vi "calc com end of volume.vi"(10 "end of volume":bool, 11 "running sums in":T1) -> (0 "ready for input":bool, 1 "output valid":bool, 2 "center of mass":cluster{"x avg":i16, "y avg":i16, "z avg":i16}, 3 "running sums out":T1, 5 "running sums eov":T1)   [LabVIEW 2010]
uses:
  <vilib>/rvi/FXPMathLib/FxpReciprocal/XNode/nifxpmath_Reciprocal.xnode
  <vilib>/rvi/FXPMathLib/FxpDiv/XNode/nifxpmath_Div.xnode
  <vilib>/rvi/FXPMathLib/FxpDiv/subVIs/nifxpmath_Div_SimConfig.ctl
  <vilib>/rvi/FXPMathLib/FxpMul/XNode/nifxpmath_Multiplier.xnode
  <vilib>/rvi/FXPMathLib/FxpMul/subVIs/nifxpmath_Mul_SimConfig.ctl
  <vilib>/fxp/LVFixedPointQuantizationPolicyTypeDef.ctl
  <vilib>/fxp/LVFixedPointOverflowPolicyTypeDef.ctl
  <vilib>/rvi/FXPMathLib/FxpDiv/simVIs/DllFxpDivTemp_sub.vi
  <vilib>/rvi/FXPMathLib/FxpMul/simVIs/DllFxpMulTemp_sub.vi
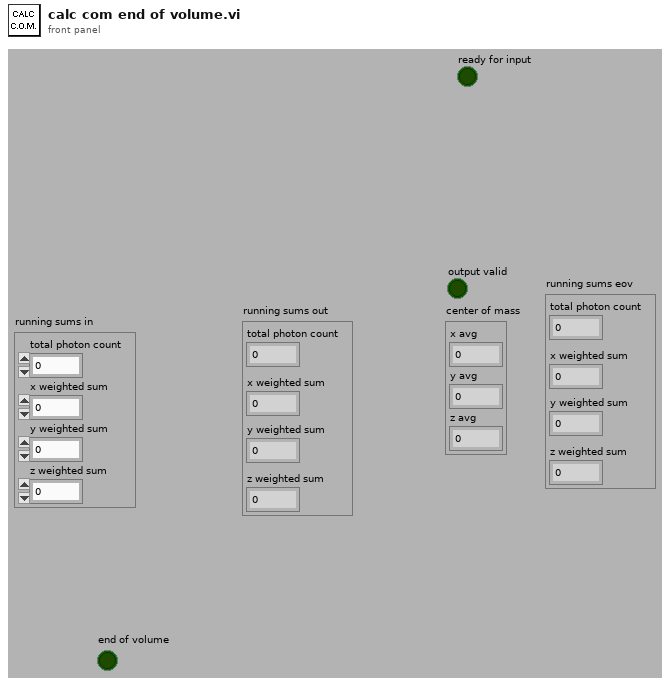
[diagram p1: front panel]
types:
  T1 = cluster{"total photon count":u64, "x weighted sum":i64, "y weighted sum":i64, "z weighted sum":i64}
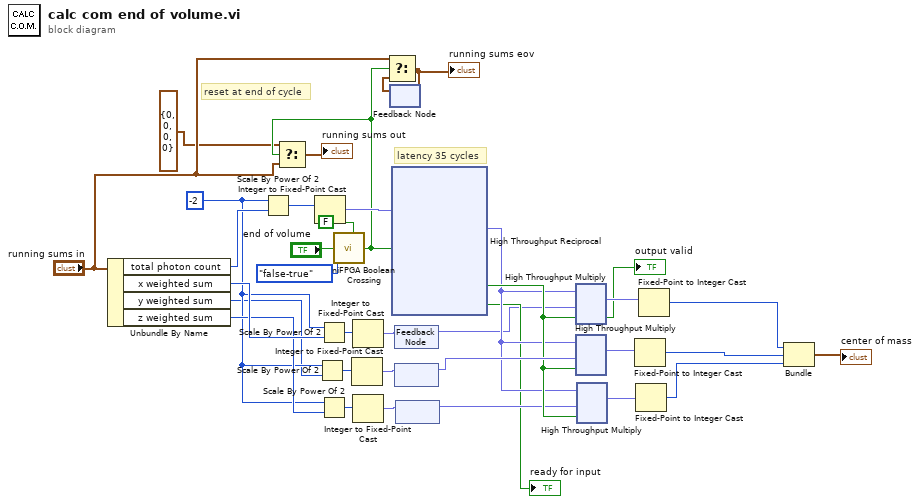
[diagram p0: block diagram]
diagram:
  w2 = -2 ("n")
  # "reset at end of cycle"
  # "latency 35 cycles"
  n1 = Unbundle By Name("running sums in") -> ("total photon count"=w9:u64, "x weighted sum"=w8:i64, "y weighted sum"=w1:i64, "z weighted sum"=w7:i64)
  n2 = Scale By Power Of 2(n=w2, x=w9) -> (x*2^n=w6:u64)
  n3 = Integer to Fixed-Point Cast(integer=w6) -> (fixed-point=w36:fxp<+,64,64>)  [unwired: 1 in]
  n4 = Scale By Power Of 2(n=w2, x=w1) -> (x*2^n=w4:i64)
  n5 = Scale By Power Of 2(n=w2, x=w8) -> (x*2^n=w5:i64)
  n6 = Scale By Power Of 2(n=w2, x=w7) -> (x*2^n=w3:i64)
  n7 = call <vilib>:"niFPGA Boolean Crossing.vi"("input"="end of volume", "direction"=enum8{"either", "false-true", "true-false"}."false-true", "initialize"=FALSE) -> ("crossing"=w13:bool)  [unwired: 6 in]
  n8 = Select(t=T1 {"total photon count"=0, "x weighted sum"=0, "y weighted sum"=0, "z weighted sum"=0} ("running sums in"), s=w13, f="running sums in") -> (s? t:f=→"running sums out":T1)
  n9 = Integer to Fixed-Point Cast(integer=w4) -> (fixed-point=w32:fxp<+/-,64,64>)  [unwired: 1 in]
  n10 = Integer to Fixed-Point Cast(integer=w5) -> (fixed-point=w17:fxp<+/-,64,64>)  [unwired: 1 in]
  n11 = Integer to Fixed-Point Cast(integer=w3) -> (fixed-point=w31:fxp<+/-,64,64>)  [unwired: 1 in]
  n12 = feedback #1() -> (w11:T1)  [unwired: 1 in]
  n13 = Select(t="running sums in", s=w13, f=w11) -> (s? t:f=w12:T1)
  "running sums eov" <- w12
  n14 = feedback-in #1(w12) -> ()
  n15 = xnode "High Throughput Reciprocal"("x"=w36, "input valid"=w13) -> ("1/x"=w27:fxp<+,32,0>, "output valid"=w29:bool, "ready for input"=→"ready for input":bool)  [unwired: 1 in]
  n16 = feedback-in #2(w17) -> ()
  n17 = feedback #2() -> (w16:fxp<+/-,64,64>)  [unwired: 1 in]
  n18 = feedback #3() -> (w30:fxp<+/-,64,64>)  [unwired: 1 in]
  n19 = feedback-in #3(w32) -> ()
  n20 = feedback #4() -> (w28:fxp<+/-,64,64>)  [unwired: 1 in]
  n21 = feedback-in #4(w31) -> ()
  n22 = xnode "High Throughput Multiply"("x"=w27, "y"=w16, "input valid"=w29) -> ("x*y"=w26:fxp<+/-,16,16>, "output valid"=→"output valid":bool)  [unwired: 1 in, 1 out]
  n23 = xnode "High Throughput Multiply"("x"=w27, "y"=w30, "input valid"=w29) -> ("x*y"=w25:fxp<+/-,16,16>)  [unwired: 1 in, 2 out]
  n24 = xnode "High Throughput Multiply"("x"=w27, "y"=w28, "input valid"=w29) -> ("x*y"=w24:fxp<+/-,16,16>)  [unwired: 1 in, 2 out]
  n25 = Fixed-Point to Integer Cast(1:w25) -> (0:w20:i16)
  n26 = Fixed-Point to Integer Cast(1:w24) -> (0:w19:i16)
  n27 = Fixed-Point to Integer Cast(1:w26) -> (0:w21:i16)
  n28 = Bundle(w21, w20, w19) -> (→"center of mass":cluster{i16, i16, i16})  [unwired: 1 in]
